vi "get.all.tests.directories.vi"(8 "error in":errorcluster, 10 "filter(s)":string[](array[string])=["hostToFpgaTests"], 11 "Path.in":path) -> (0 "error out":errorcluster, 3 "Test Directories":path[](array[path]))   [LabVIEW 2020, in "fpganow.common.host.lvlib"]
uses:
  fpganow.common.host.lvlib
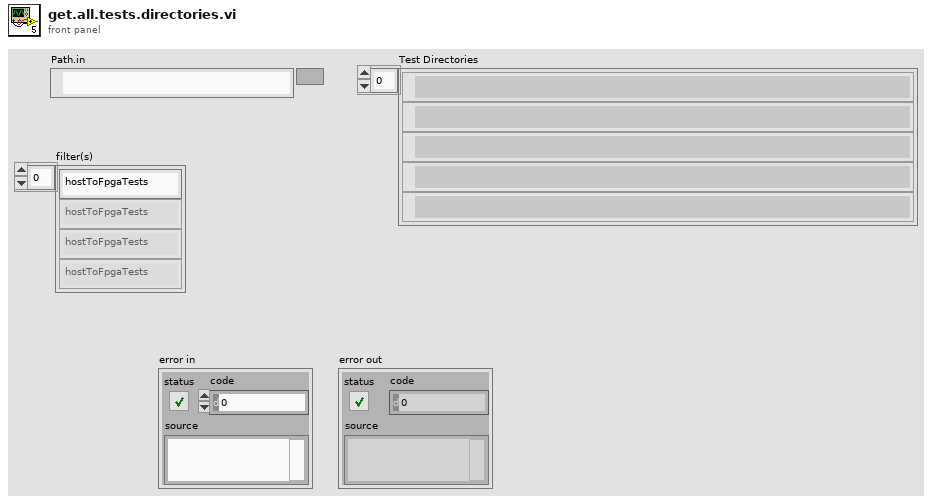
[diagram p1: front panel]
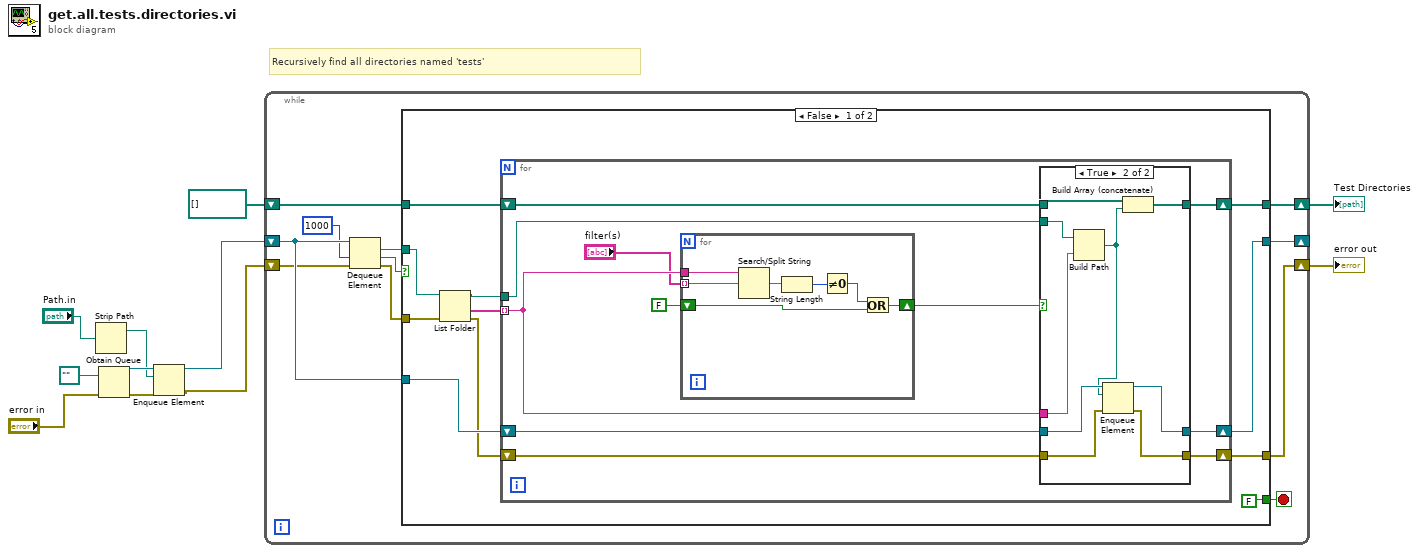
[diagram p0: block diagram]
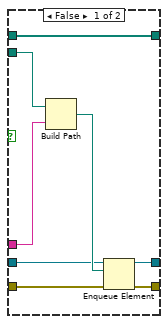
[diagram p2: hidden frame]
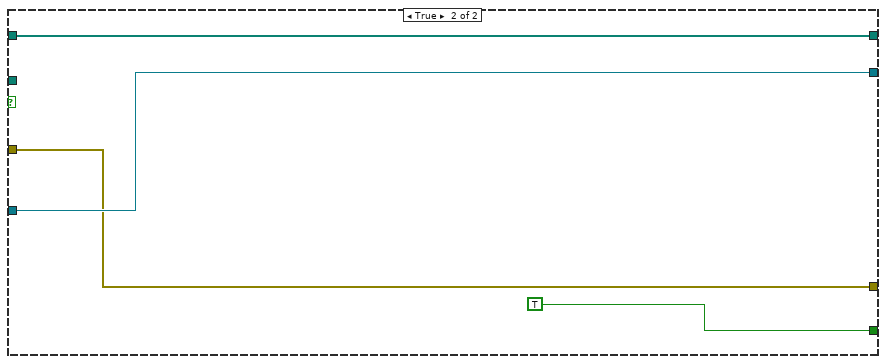
[diagram p3: hidden frame]
diagram:
  # "Recursively find all directories named 'tests'"
  n1 = Strip Path(path="Path.in") -> (stripped path=w8:path)  [unwired: 1 out]
  n2 = Obtain Queue(element data type=path "" ("stripped path"), error in (no error)="error in") -> (queue out=w9:refnum<queue>, error out=w3:errorcluster)  [unwired: 3 in, 1 out]
  n3 = Enqueue Element(queue=w9, element=w8, error in (no error)=w3) -> (queue out=w6:refnum<queue>, error out=w2:errorcluster)  [unwired: 1 in, 1 out]
  n4 = while {
    shift-right: [w22] -> w11
    shift-left: path[] [] -> [w20]
    shift-right: [w17] -> _
    shift-left: w6 -> [w16]
    shift-right: [w12] -> w1
    shift-left: w2 -> [w14]
    stop <- w18 stop-if-true
    n5 = Dequeue Element(queue=w16, timeout in ms (-1)=1000, error in (no error)=w14) -> (element=w21:path, timed out?=w19:bool, error out=w13:errorcluster)  [unwired: 1 out]
    n6 = case shown="False" w19 {
      tunnel: [w32 w71] -> w22
      tunnel: w21 -> [w30 _]
      tunnel: w20 -> [w29 w71]
      tunnel: [FALSE TRUE] -> w18
      tunnel: [w26 w70] -> w17
      tunnel: w16 -> [w27 w70]
      tunnel: w13 -> [w25 w69]
      tunnel: [w23 w69] -> w12
      frame False {
        n7 = List Folder(path=w30, error in=w25) -> (path out=w31:path, folder names=w33:string[], error out=w24:errorcluster)  [unwired: 2 in, 1 out]
        n8 = for {
          tunnel: w33 -> [w37] mode=indexing
          shift-right: [w43] -> w32
          shift-left: w29 -> [w44]
          tunnel: w31 -> [w42]
          shift-right: [w40] -> w26
          shift-left: w27 -> [w41]
          shift-right: [w38] -> w23
          shift-left: w24 -> [w39]
          n9 = for {
            tunnel: w37 -> [w49]
            tunnel: "filter(s)" -> [w50] mode=indexing
            shift-right: [w45] -> w34
            shift-left: FALSE -> [w51]
            n10 = Search/Split String(string=w49, search string/char (-)=w50) -> (match + rest of string=w48:string)  [unwired: 1 in, 2 out]
            n11 = String Length(string=w48) -> (length=w47:i32)
            n12 = Not Equal To 0?(x=w47) -> (x != 0?=w46:bool)
            n13 = Or(x=w46, y=w51) -> (x .or. y?=w45:bool)
          }
          n14 = case shown="True" w34 {
            tunnel: w44 -> [w59 w68]
            tunnel: [w59 w67] -> w43
            tunnel: w42 -> [w58 w66]
            tunnel: w41 -> [w56 w64]
            tunnel: [w55 w63] -> w40
            tunnel: w37 -> [w54 w65]
            tunnel: w39 -> [w53 w61]
            tunnel: [w52 w62] -> w38
            frame False {
              n15 = Build Path(base path=w58, name or relative path=w54) -> (appended path=w57:path)
              n16 = Enqueue Element(queue=w56, element=w57, error in (no error)=w53) -> (queue out=w55:refnum<queue>, error out=w52:errorcluster)  [unwired: 1 in, 1 out]
            }
            frame True {
              n17 = Build Path(base path=w66, name or relative path=w65) -> (appended path=w60:path)
              n18 = Enqueue Element(queue=w64, element=w60, error in (no error)=w61) -> (queue out=w63:refnum<queue>, error out=w62:errorcluster)  [unwired: 1 in, 1 out]
              n19 = Build Array (concatenate)(w68, w60) -> (w67:path[])
            }
          }
        }
      }
      frame True {
      }
    }
  }
  "Test Directories" <- w11
  "error out" <- w1
